vi "Set Filter.vi"(8 "error in (no error)":errorcluster, 10 "Filters":T1(ring), 11 "data":waveform(dbl)[](array[waveform])) -> (0 "error out":errorcluster, 3 "Array of Waveform":waveform(dbl)[](array[waveform]))   [LabVIEW 2017]
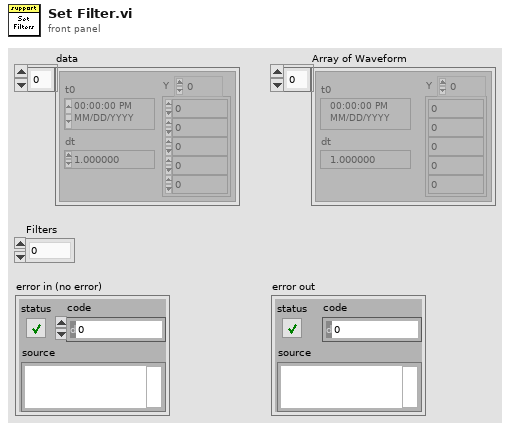
[diagram p1: front panel]
types:
  T1 = enum16{"0", "0.1", "0.2", "0.5", "1", "2", "5", "10", "20", "50", "100", "200", "500", "1000", "2000", "5000", "10000"}
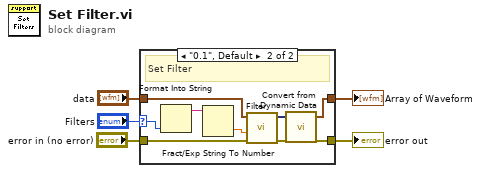
[diagram p0: block diagram]
diagram:
  n1 = case shown="\"0.1\", Default" "Filters" {
    selector: "Filters" -> [_ w10]
    tunnel: "data" -> [w7 w15]
    tunnel: "error in (no error)" -> [w6 w13]
    tunnel: [w6 w12] -> w2
    tunnel: [w7 w11] -> w4
    frame "0" {
    }
    frame "0.1", Default {
      # "Set Filter"
      n2 = Format Into String(w10) -> (resulting string=w9:string)  [unwired: 3 in, 1 out]
      n3 = Fract/Exp String To Number(string=w9) -> (number=w8:dbl)  [unwired: 3 in, 1 out]
      n4 = call "Filter"("error in (no error)"=w13, "Lower Cut-Off"=w8, "Signal"=w15) -> ("error out"=w12:errorcluster, "Filtered Signal"=w14:dynamicdata)  [unwired: 7 in]
      n5 = call "Convert from Dynamic Data"("Dynamic Data Type"=w14) -> ("Array of Waveform"=w11:waveform(dbl)[])  [unwired: 3 in]
    }
  }
  "Array of Waveform" <- w4
  "error out" <- w2
